vi "Error Query.vi"(8 "error in (no error)":errorcluster, 11 "VISA resource name":refnum<visa-resource-name>) -> (0 "error out":errorcluster, 1 "Error Message":string, 2 "Error Code":i32[](array[numeric]), 3 "VISA resource name out":refnum<visa-resource-name>)   [LabVIEW 2017, in "Scope.lvlib" / "Tektronix DPO MSO 2000 4000 Series.lvlib"]
doc: "Queries an instrument for any errors in the error queue of the instrument. The Error Query VI continuously reads errors until this VI reads all the errors from the instrument. \n<B>Note</B>: Because most driver VIs automatically call the Error Query VI, you do not need to call this VI in an application."
uses:
  Tektronix DPO MSO 2000 4000 Series.lvlib
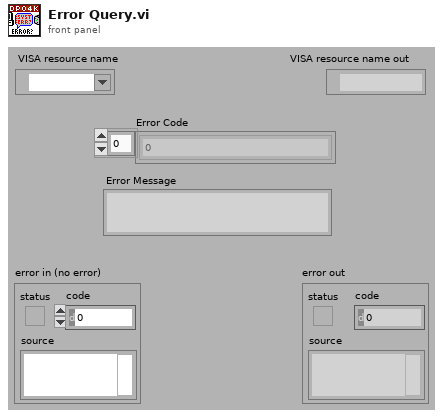
[diagram p1: front panel]
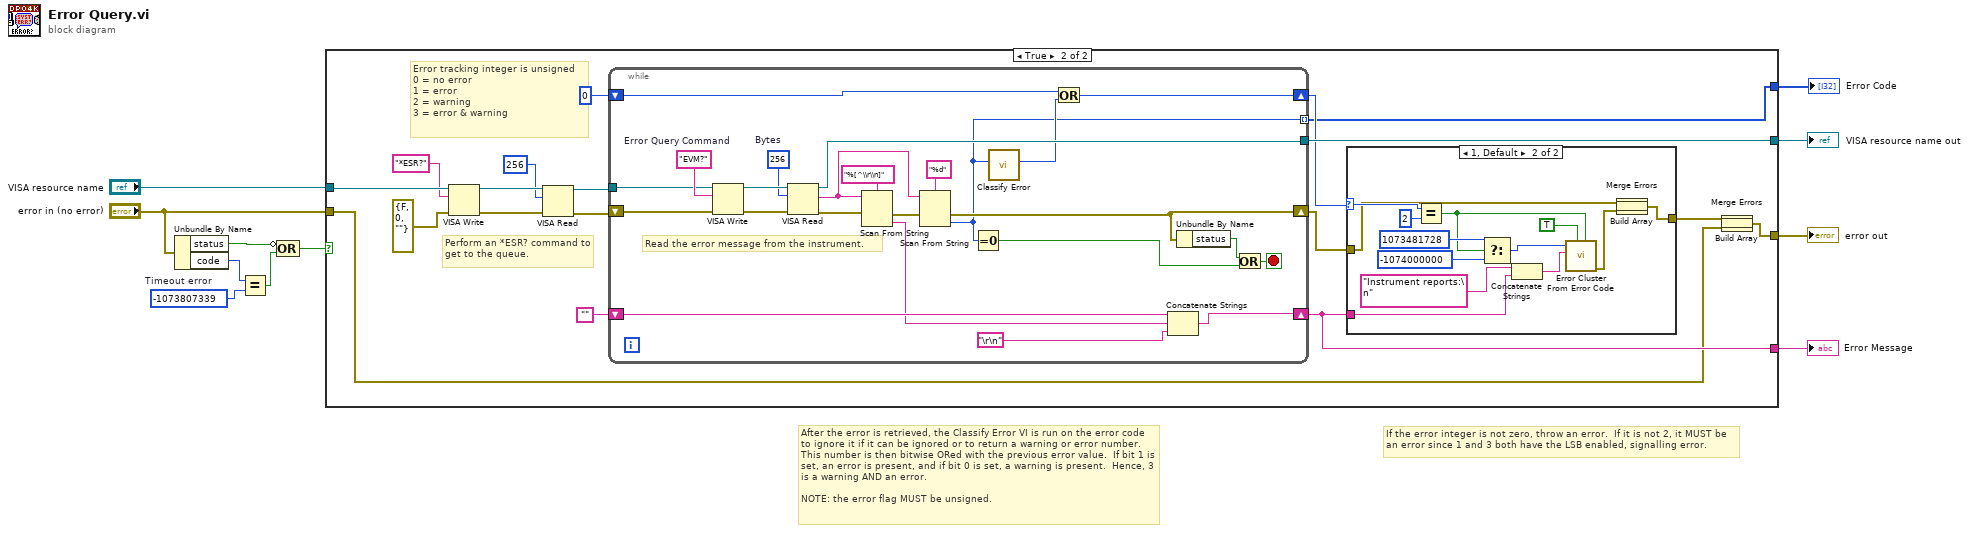
[diagram p0: block diagram]
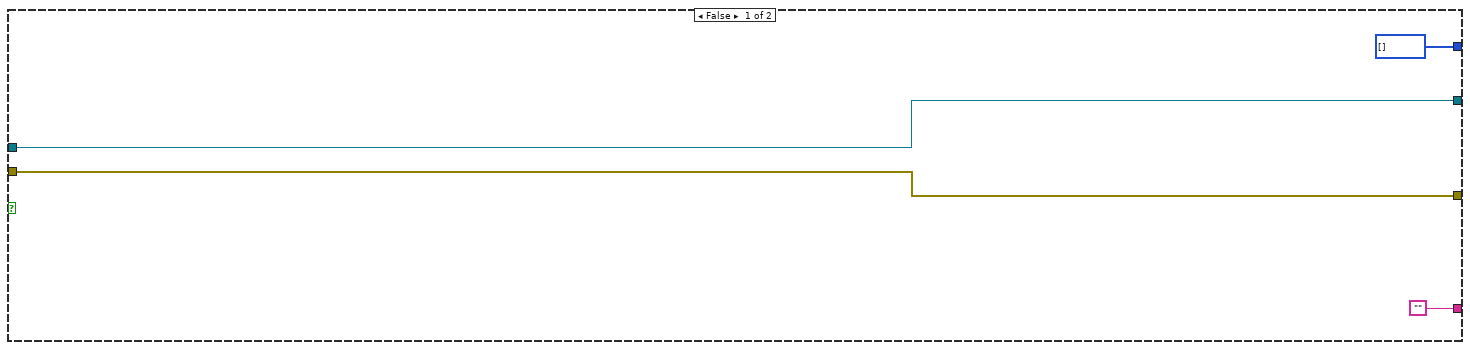
[diagram p2: hidden frame]
diagram:
  w6 = -1073807339  # Timeout error
  # "If the error integer is not zero, throw an error.  If it is not 2, it MUST be an error since 1 and 3 both have the LSB enabled, signalling error."
  # "After the error is retrieved, the Classify Error VI is run on the error code to ignore it if it can be ignored or to return a warning or error number.  This number is then bitwise ORed with the previous error value.  If bit 1 is set, an error is present, and if bit 0 is set, a warning is present.  Hence, 3 is a warning AND an error.\n\nNOTE: the error flag MUST be unsigned."
  n1 = Unbundle By Name("error in (no error)") -> ("status"=w7:bool, "code"=w4:i32)
  n2 = Equal?(x=w4, y=w6) -> (x = y?=w5:bool)
  n3 = Compound Arithmetic op=OR(invert w7, w5) -> (w3:bool)
  n4 = case shown="True" w3 {
    tunnel: [w15 w34] -> w11
    tunnel: "VISA resource name" -> [w15 w30]
    tunnel: "error in (no error)" -> [w14 w17]
    tunnel: [w14 w32] -> w9
    tunnel: ["" w31] -> w2
    tunnel: [i32[] [] w19] -> w1
    frame False {
    }
    frame True {
      # "Error tracking integer is unsigned\n0 = no error\n1 = error\n2 = warning\n3 = error & warning"
      # "Perform an *ESR? command to get to the queue."
      n5 = VISA Write(VISA resource name=w30, write buffer="*ESR?", error in (no error)=errorcluster {"status"=FALSE, "code"=0, "source"=""}) -> (VISA resource name out=w27:refnum<visa-resource-name>, error out=w28:errorcluster)  [unwired: 1 out]
      n6 = VISA Read(VISA resource name=w27, byte count=u32 256, error in (no error)=w28) -> (VISA resource name out=w25:refnum<visa-resource-name>, error out=w24:errorcluster)  [unwired: 2 out]
      n7 = while {
        tunnel: [w73] -> w34
        tunnel: w25 -> [w56]
        shift-right: [w62] -> w31
        shift-left: "" -> [w64]
        shift-right: [w53] -> w22
        shift-left: u32 0 ("x = 0?") -> [w52]
        shift-right: [w60] -> w21
        shift-left: w24 -> [w61]
        tunnel: [w50] -> w19 mode=indexing
        stop <- w67 stop-if-true
        w71 = u32 256  # Bytes
        w69 = "EVM?"  # Error Query Command
        # "Read the error message from the instrument."
        n8 = VISA Write(VISA resource name=w56, write buffer=w69, error in (no error)=w61) -> (VISA resource name out=w72:refnum<visa-resource-name>, error out=w70:errorcluster)  [unwired: 1 out]
        n9 = VISA Read(VISA resource name=w72, byte count=w71, error in (no error)=w70) -> (VISA resource name out=w73:refnum<visa-resource-name>, read buffer=w65:string, error out=w59:errorcluster)  [unwired: 1 out]
        n10 = Scan From String(format string="%[^\\r\\n]", input string=w65, error in=w59) -> (error out=w58:errorcluster, output 1=w63:string)  [unwired: 2 in, 2 out]
        n11 = Scan From String(format string="%d", input string=w65, error in=w58) -> (error out=w60:errorcluster, output 1=w50:i32)  [unwired: 2 in, 2 out]
        n12 = Equal To 0?(x=w50) -> (x = 0?=w55:bool)
        n13 = call "Classify Error.vi"("Error Code"=w50) -> ("Error Classification"=w51:i32)  [unwired: 10 in]
        n14 = Or(x=w52, y=w51) -> (x .or. y?=w53:u32)
        n15 = Concatenate Strings(w64, w63, "\r\n") -> (w62:string)
        n16 = Unbundle By Name(w60) -> ("status"=w57:bool)
        n17 = Or(x=w57, y=w55) -> (x .or. y?=w67:bool)
      }
      n18 = case shown="1, Default" w22 {
        selector: w22 -> [_ w45]
        tunnel: [w35 w37] -> w18
        tunnel: w31 -> [_ w46]
        tunnel: w21 -> [w35 w39]
        frame 0 {
        }
        frame 1, Default {
          n19 = Equal?(x=w45, y=u32 2) -> (x = y?=w42:bool)
          n20 = Select(t=1073481728 ("Code"), s=w42, f=-1074000000 ("Code")) -> (s? t:f=w40:i32)
          n21 = Concatenate Strings("Instrument reports:\n" ("Source"), w46) -> (w47:string)
          n22 = call <vilib>:"Error Cluster From Error Code.vi"("is warning? (False)"=w42, "show call chain? (False)"=TRUE, "error message (\"\")"=w47, "error code (0)"=w40) -> ("error out"=w38:errorcluster)  [unwired: 5 in]
          n23 = Build Array(w39, w38) -> (w36:errorcluster[])
          n24 = Merge Errors(w36) -> (w37:errorcluster)
        }
      }
      n25 = Build Array(w18, w17) -> (w16:errorcluster[])
      n26 = Merge Errors(w16) -> (w32:errorcluster)
    }
  }
  "VISA resource name out" <- w11
  "error out" <- w9
  "Error Message" <- w2
  "Error Code" <- w1
